vi "init.vi"(0 "+3.3VASupplyTest in":refnum<class "+3.3VASupplyTest.lvclass">, 1 "Log":refnum<class "ITestLog.lvclass">, 5 "DAQ Channel To Read":refnum<k21>, 7 "Expected Value":dbl[unit], 9 "Tolerance":dbl[unit], 11 "error in (no error)":errorcluster, 12 "Samples To Read":dbl) -> (4 "+3.3VASupplyTest out":refnum<class "+3.3VASupplyTest.lvclass">, 15 "error out":errorcluster)   [LabVIEW 2015, in "+3.3VASupplyTest.lvclass"]
uses:
  +3.3VASupplyTest.lvclass
  Model/TestLog/ITestLog/ITestLog.lvclass
  +3.3VASupplyTest.lvclass/+3.3VASupplyTest.ctl
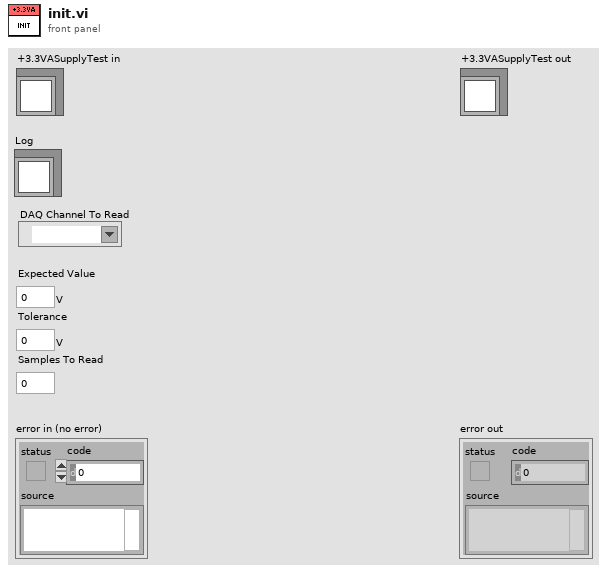
[diagram p1: front panel]
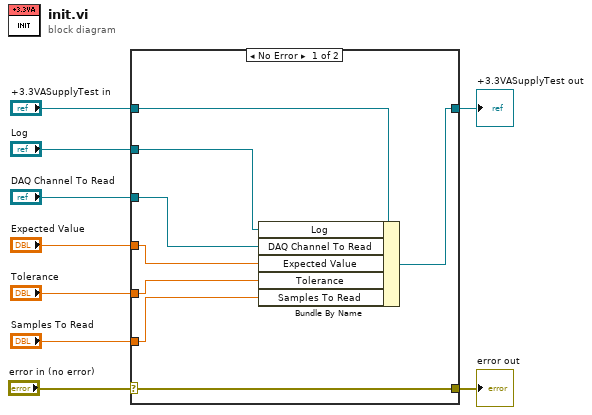
[diagram p0: block diagram]
diagram:
  n1 = case shown="No Error" "error in (no error)" {
    selector: "error in (no error)" -> [w17 w19]
    tunnel: [w17 w19] -> w8
    tunnel: [w15 w18] -> w6
    tunnel: "+3.3VASupplyTest in" -> [w16 w18]
    tunnel: "Log" -> [w10 _]
    tunnel: "DAQ Channel To Read" -> [w11 _]
    tunnel: "Expected Value" -> [w12 _]
    tunnel: "Tolerance" -> [w13 _]
    tunnel: "Samples To Read" -> [w14 _]
    frame No Error {
      n2 = Bundle By Name(cluster=w16, "Log"=w10, "DAQ Channel To Read"=w11, "Expected Value"=w12, "Tolerance"=w13, "Samples To Read"=w14) -> (w15:refnum<class "+3.3VASupplyTest.lvclass">)
    }
    frame Error {
    }
  }
  "error out" <- w8
  "+3.3VASupplyTest out" <- w6
